vi "api_get_openweather.vi"(8 "error in":errorcluster, 10 "Key Value Query":string[][](table)=[["zip", "80004,us"], ["units", "imperial"], ["appid", "73bd1b5172624640c9af2d8fa6381cf4"]], 11 "client handle":T2) -> (0 "error out":errorcluster, 2 "Cluster Out":T1, 3 "client handle out":T2)   [LabVIEW 2020]
doc: "API Call to OpenWeatherMap.org. URL and parameters already provided. Key Value Query can be changed for different information. Unbundle output cluster to get data."
uses:
  <vilib>/httpClient/ClientHandle.ctl
  <vilib>/httpClient/LabVIEWHTTPClient.lvlib
panel:
  in  "Base URL":string="api.openweathermap.org/data/2.5/weather?"
  out "Full URL":string
  out "body":string
  out "headers":string
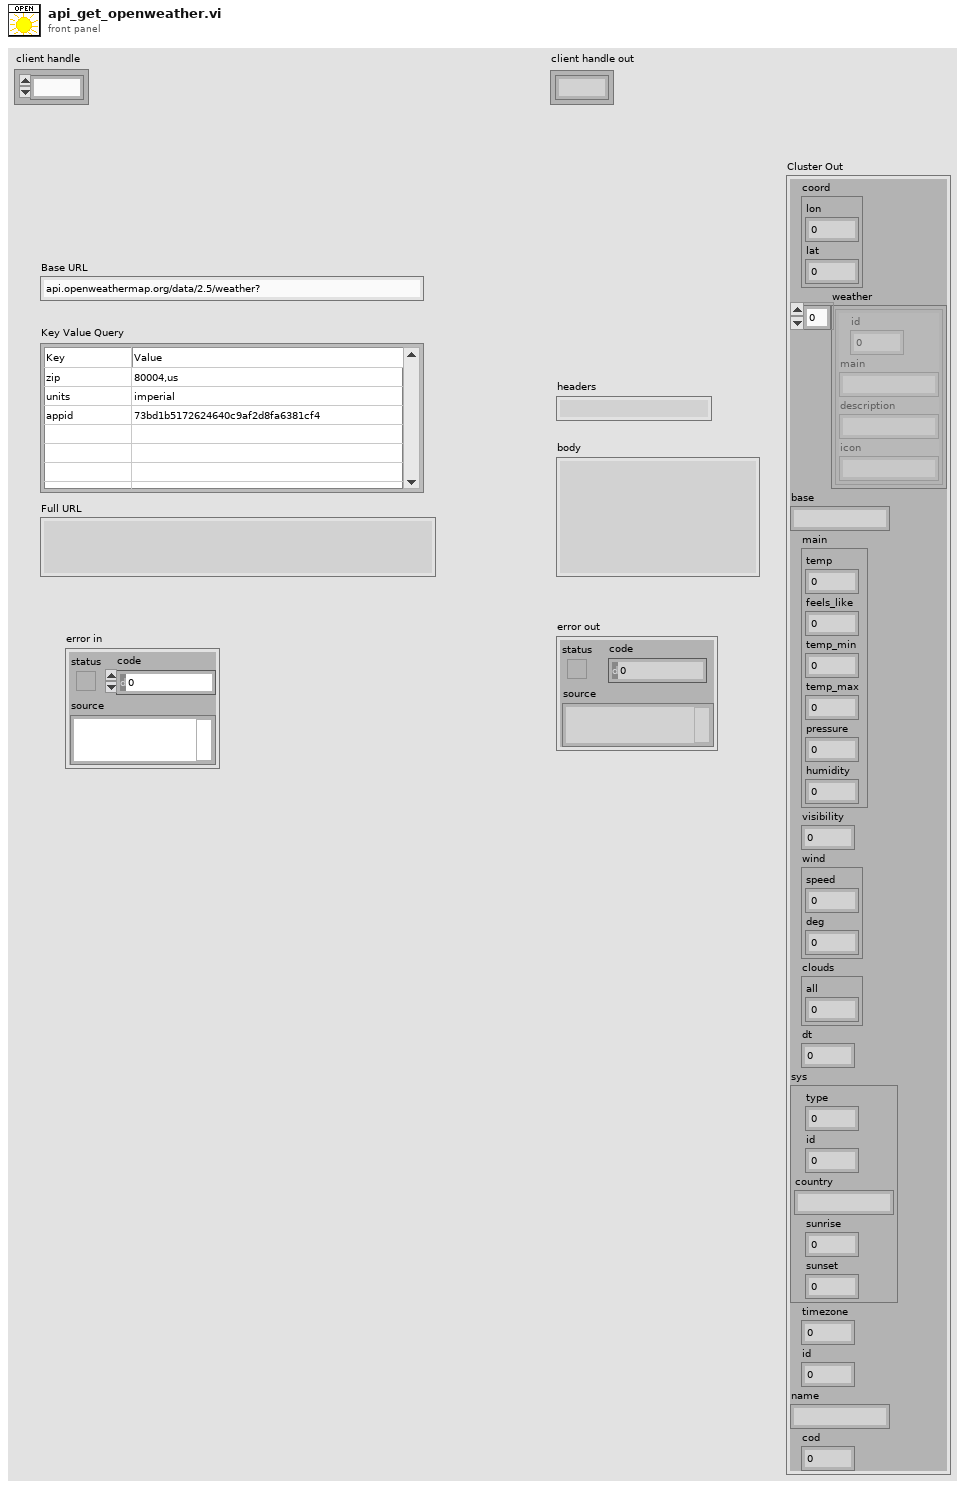
[diagram p1: front panel]
types:
  T1 = cluster{"coord":cluster{"lon":dbl, "lat":dbl}, "weather":cluster{"id":i32, "main":string, "description":string, "icon":string}[], "base":string, "main":cluster{"temp":dbl, "feels_like":dbl, "temp_min":dbl, "temp_max":dbl, "pressure":dbl, "humidity":dbl}, "visibility":i32, "wind":cluster{"speed":i32, "deg":i32}, "clouds":cluster{"all":i32}, "dt":i32, "sys":cluster{"type":i32, "id":i32, "country":string, "sunrise":i32, "sunset":i32}, "timezone":i32, "id":i32, "name":string, "cod":i32}
  T2 = typedef "LabVIEWHTTPClient.lvlib/ClientHandle.ctl" = refnum<k1>
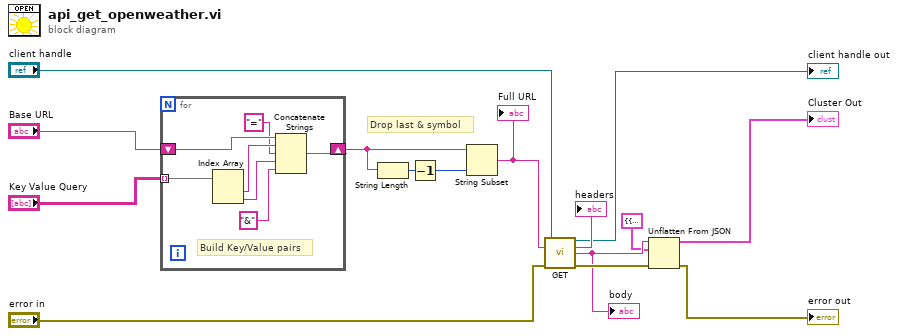
[diagram p0: block diagram]
diagram:
  # "Drop last & symbol"
  n1 = for {
    tunnel: "Key Value Query" -> [w22] mode=indexing
    shift-right: [w17] -> w5
    shift-left: "Base URL" -> [w21]
    # "Build Key/Value pairs"
    n2 = Index Array(array=w22) -> (element #1=w20:string, element #2=w18:string)  [unwired: 2 in]
    n3 = Concatenate Strings(w21, w20, "=" ("string"), w18, "&" ("string")) -> (w17:string)
  }
  n4 = String Length(string=w5) -> (length=w7:i32)
  n5 = Decrement(x=w7) -> (x-1=w6:i32)
  n6 = String Subset(string=w5, length (rest)=w6) -> (substring=w4:string)  [unwired: 1 in]
  "Full URL" <- w4
  n7 = call <vilib>:"GET.vi"("client handle"="client handle", "url"=w4, "error in (no error)"="error in") -> ("client handle out"=→"client handle out":T2, "headers"=→"headers":string, "body"=w12:string, "error out"=w13:errorcluster)  [unwired: 9 in]
  "body" <- w12
  n8 = Unflatten From JSON(JSON string=w12, type and defaults=T1 {"coord"={"lon"=0.0, "lat"=0.0}, "weather"=[{"id"=0, "main"="", "description"="", "icon"=""}, {"id"=0, "main"="", "description"="", "icon"=""}], "base"="", "main"={"temp"=0.0, "feels_like"=0.0, "temp_min"=0.0, "temp_max"=0.0, "pressure"=0.0, "humidity"=0.0}, "visibility"=0, "wind"={"speed"=0, "deg"=0}, "clouds"={"all"=0}, "dt"=0, "sys"={"type"=0, "id"=0, "country"="", "sunrise"=0, "sunset"=0}, "timezone"=0, "id"=0, "name"="", "cod"=0} ("Cluster"), error in (no error)=w13) -> (value=→"Cluster Out":T1, error out=→"error out":errorcluster)  [unwired: 4 in]
